vi "Get Tool Config Cluster Version.vi"() -> (3 "Config Cluster Version":string)   [LabVIEW 2015, in "Tool Cfg.lvlib"]
uses:
  Tool Cfg.lvlib
  ConfigGLOB.vi
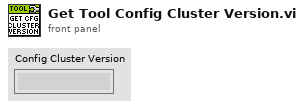
[diagram p1: front panel]
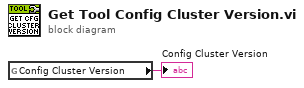
[diagram p0: block diagram]
diagram:
  n1 = global read "ConfigGLOB.vi" "Config Cluster Version"() -> (→"Config Cluster Version":string)
